vi "Read New Send Method.vi"(11 "Concrete Send Builder in":refnum<class "Concrete Send Builder.lvclass">) -> (2 "New Send Method":path)   [LabVIEW 2020, in "Message Maker.lvlib" / "Concrete Send Builder.lvclass"]
uses:
  Concrete Send Builder.lvclass
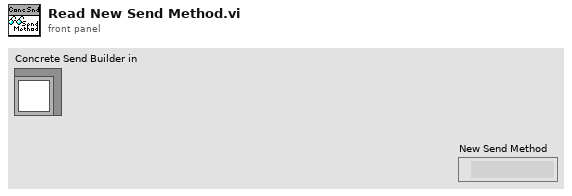
[diagram p1: front panel]
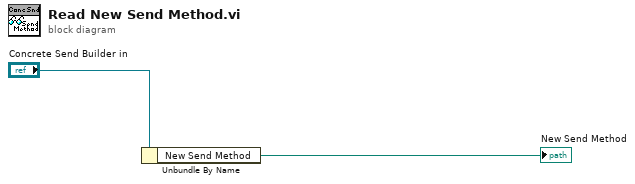
[diagram p0: block diagram]
diagram:
  n1 = Unbundle By Name("Concrete Send Builder in") -> ("New Send Method"=→"New Send Method":path)
